vi "与工控机交互(子VI).vi"   [LabVIEW 2016, in "数据传输系统.lvlib"]
uses:
  <vilib>/ptbypt/NI_PtbyPt.lvlib
types:
  T1 = cluster{"setini":string, "sysini":string, "hechaini":string, "actualwrite":string, "actualread":string, "datasent":string, "反控命令信息队列":string, "反控与仪器交互":string}
  T2 = cluster{"仪器状态":u16[], "试剂余量":u16[], "各参数测量间隔":u16[], "关键参数":u16[], "校准点信息":u16[], "告警信息":u16[], "系统信息":u16[]}
  T3 = cluster{"[0]":bool, "[1]":bool, "[2]":bool, "[3]":bool, "[4]":bool}
  T4 = cluster{"[0]":bool, "[1]":bool, "[2]":bool, "[3]":bool, "[4]":bool, "[5]":bool}
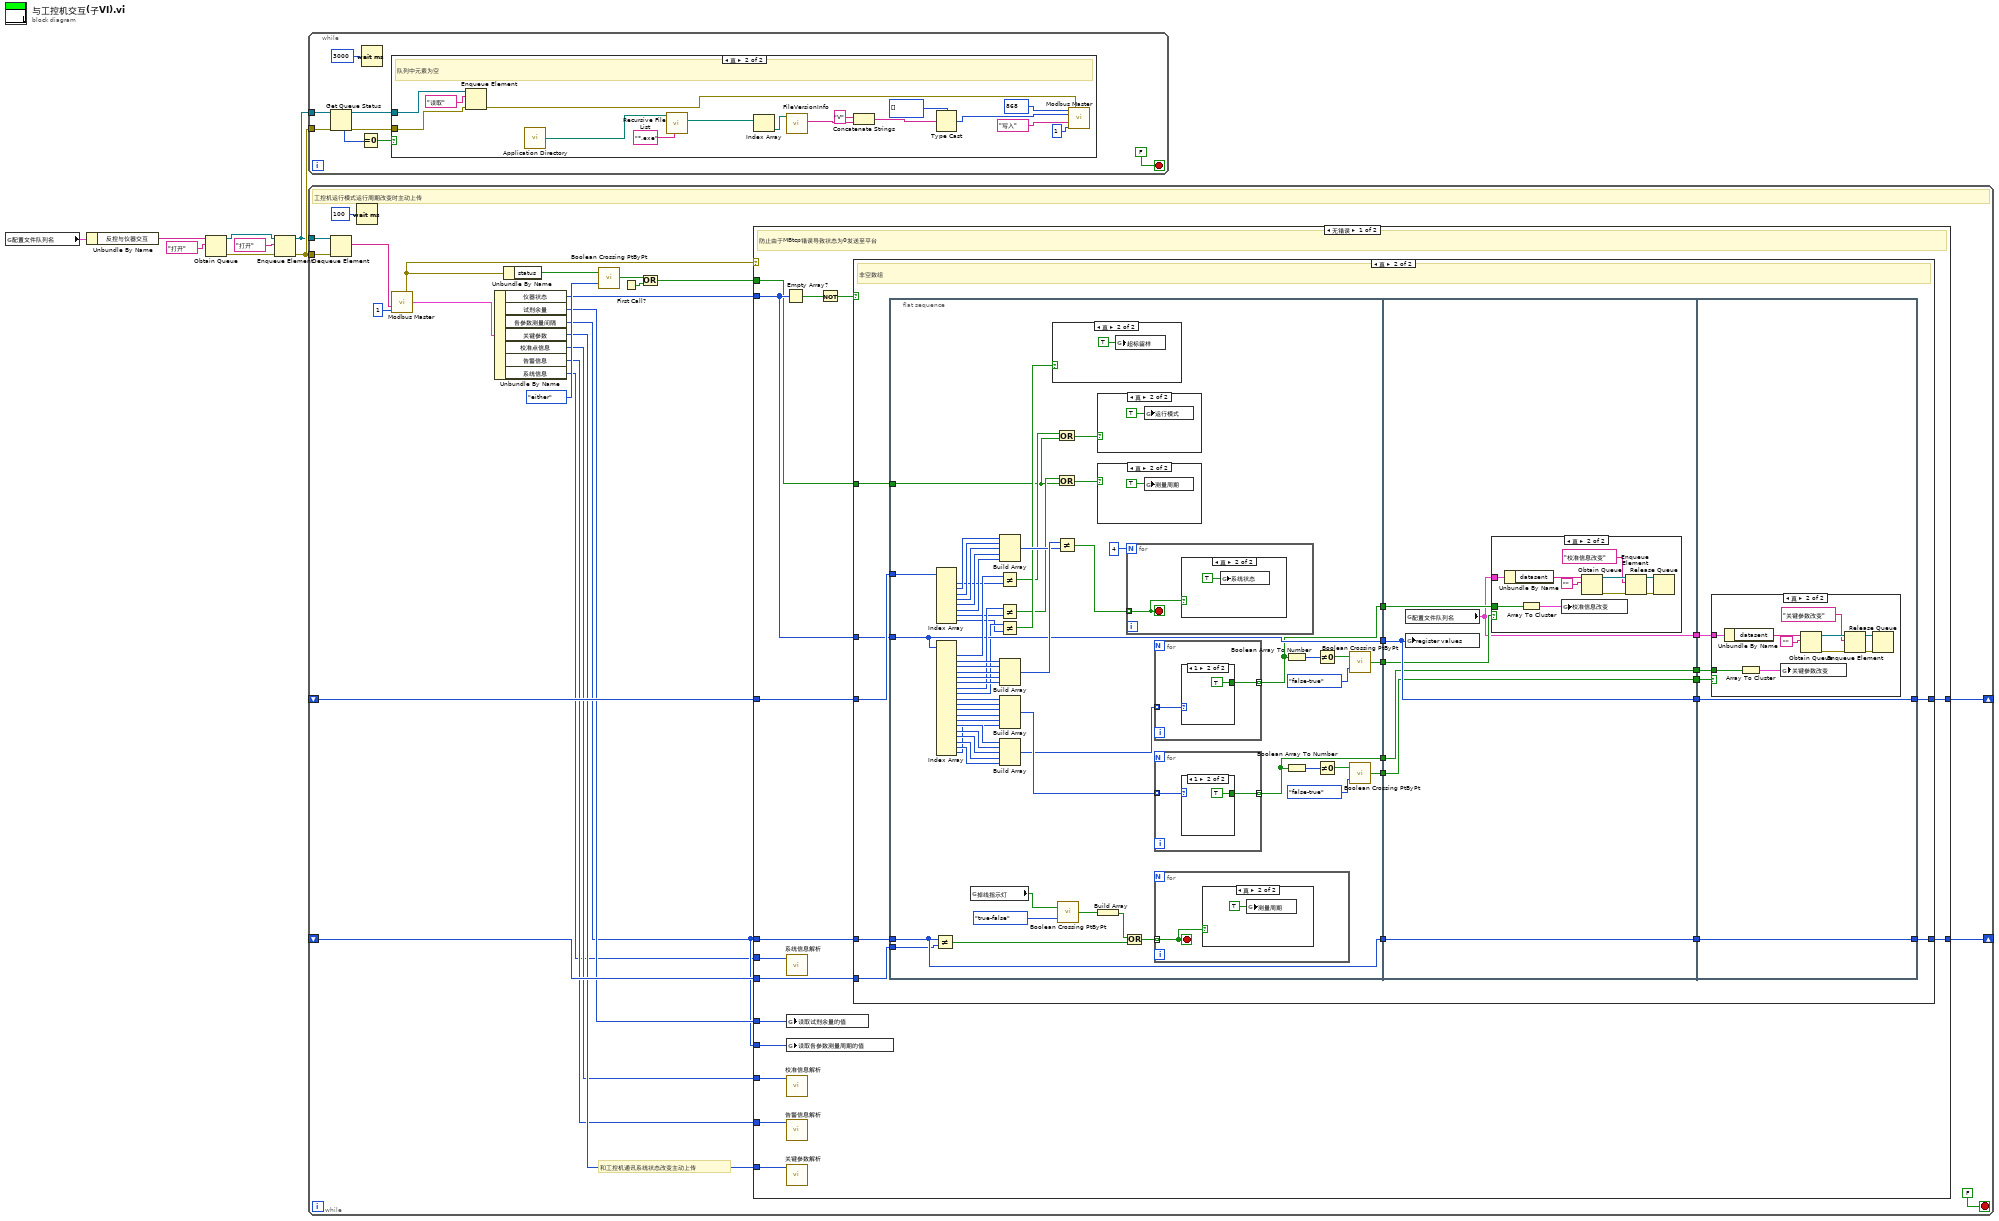
[diagram p0: block diagram]
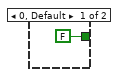
[diagram p4: hidden frame]
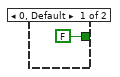
[diagram p5: hidden frame]
diagram:
  n1 = global read "全局1.vi" "配置文件队列名"() -> (w1:T1)
  n2 = Unbundle By Name(w1) -> ("反控与仪器交互"=w2:string)
  n3 = Obtain Queue(name (unnamed)=w2, element data type="打开" ("读取写入选择")) -> (queue out=w4:refnum<queue>, error out=w5:errorcluster)  [unwired: 3 in, 1 out]
  n4 = Enqueue Element(queue=w4, element="打开" ("读取写入选择"), error in (no error)=w5) -> (queue out=w6:refnum<queue>, error out=w7:errorcluster)  [unwired: 1 in, 1 out]
  n5 = while {
    tunnel: w6 -> [w13]
    tunnel: w7 -> [w12]
    stop <- FALSE stop-if-true
    n6 = Get Queue Status(queue=w13, error in (no error)=w12) -> (queue out=w10:refnum<queue>, error out=w9:errorcluster, # elements in queue=w14:i32)  [unwired: 1 in, 5 out]
    n7 = Equal To 0?(x=w14) -> (x = 0?=w11:bool)
    n8 = Wait (ms)(milliseconds to wait=u32 3000 ("等待时间（毫秒）")) -> ()  [unwired: 1 out]
    n9 = case shown="真" w11 {
      tunnel: w10 -> [_ w31]
      tunnel: w9 -> [_ w30]
      frame False {
      }
      frame True {
        # "队列中元素为空"
        n10 = Enqueue Element(queue=w31, element="读取" ("读取写入选择"), error in (no error)=w30) -> (error out=w26:errorcluster)  [unwired: 1 in, 2 out]
        n11 = call <vilib>:"Application Directory.vi"() -> ("Application Directory"=w24:path)
        n12 = call <vilib>:"Recursive File List.vi"("pattern"="*.exe", "Folder Path"=w24) -> ("All Files in Dir"=w22:path[])  [unwired: 5 in, 4 out]
        n13 = Index Array(array=w22) -> (element=w23:path)  [unwired: 1 in]
        n14 = call <vilib>:"FileVersionInfo.vi"("Application Path in"=w23) -> ("File Version Info"=w20:string)  [unwired: 7 in, 3 out]
        n15 = Concatenate Strings("V" ("字符串"), w20) -> (w18:string)
        n16 = Type Cast(type=u16[] [], x=w18) -> (*(type *) &x=w19:u16[])
        n17 = call "Modbus Master.vi"("starting address"=u16 868, "error in"=w26, "holding register values"=w19, "读取写入选择"="写入", "Unit ID"=u8 1) -> ()  [unwired: 4 in, 7 out]
      }
    }
  }
  n18 = while {
    tunnel: w6 -> [w53]
    tunnel: w7 -> [w52]
    shift-right: [w49] -> _
    shift-left: _ -> [w50]
    shift-right: [w42] -> _
    shift-left: _ -> [w41]
    stop <- FALSE stop-if-true
    # "和工控机通讯系统状态改变主动上传"
    # "工控机运行模式运行周期改变时主动上传"
    n19 = Dequeue Element(queue=w53, error in (no error)=w52) -> (element=w51:string)  [unwired: 1 in, 3 out]
    n20 = Wait (ms)(milliseconds to wait=u32 100 ("等待时间（毫秒）")) -> ()  [unwired: 1 out]
    n21 = call "Modbus Master.vi"("读取写入选择"=w51, "Unit ID"=u8 1) -> ("error out"=w48:errorcluster, "输出"=w40:T2)  [unwired: 7 in, 5 out]
    n22 = Unbundle By Name(w40) -> ("仪器状态"=w39:u16[], "试剂余量"=w38:u16[], "各参数测量间隔"=w37:u16[], "关键参数"=w36:u16[], "校准点信息"=w35:u16[], "告警信息"=w34:u16[], "系统信息"=w33:u16[])
    n23 = Unbundle By Name(w48) -> ("status"=w47:bool)
    n24 = call <vilib>:"Boolean Crossing PtByPt.vi"("direction"=enum16{"either", "false-true", "true-false"}."either", "input"=w47) -> ("crossing"=w45:bool)  [unwired: 1 in]
    n25 = First Call?() -> (First Call?: T/F=w44:bool)
    n26 = Or(x=w45, y=w44) -> (x .or. y?=w43:bool)
    n27 = case shown="无错误" w48 {
      tunnel: w39 -> [w69 _]
      tunnel: w50 -> [w71 w199]
      tunnel: [w70 w199] -> w49
      tunnel: w43 -> [w66 _]
      tunnel: w38 -> [w65 _]
      tunnel: w37 -> [w64 _]
      tunnel: w37 -> [w63 w198]
      tunnel: [w62 w198] -> w42
      tunnel: w41 -> [w61 _]
      tunnel: w36 -> [w60 _]
      tunnel: w35 -> [w59 _]
      tunnel: w34 -> [w58 _]
      tunnel: w33 -> [w57 _]
      frame No Error {
        # "防止由于MBtcp错误导致状态为0发送至平台"
        n28 = Empty Array?(array=w69) -> (empty?=w68:bool)
        n29 = call "系统信息解析.vi"("系统信息"=w57) -> ()  [unwired: 11 in]
        n30 = global write "全局1.vi" "读取试剂余量的值"(w65) -> ()
        n31 = global write "全局1.vi" "读取各参数测量周期的值"(w64) -> ()
        n32 = call "校准信息解析.vi"("校准信息"=w59) -> ()  [unwired: 11 in]
        n33 = call "告警信息解析.vi"("告警信息"=w58) -> ()  [unwired: 11 in]
        n34 = call "关键参数解析.vi"("关键参数"=w60) -> ()  [unwired: 11 in]
        n35 = Not(x=w68) -> (.not. x?=w67:bool)
        n36 = case shown="真" w67 {
          tunnel: w71 -> [w73 w90]
          tunnel: [w73 w89] -> w70
          tunnel: w69 -> [_ w88]
          tunnel: w66 -> [_ w87]
          tunnel: w63 -> [w72 w86]
          tunnel: [w72 w84] -> w62
          tunnel: w61 -> [_ w83]
          frame False {
          }
          frame True {
            # "非空数组"
            n37 = flat-sequence {
              tunnel: w88 -> [w134]
              tunnel: [w134] -> w91
              tunnel: w90 -> [w130]
              tunnel: w87 -> [w125]
              tunnel: w86 -> [w123]
              tunnel: [w123] -> w85
              tunnel: w83 -> [w122]
              tunnel: [w111] -> w82
              tunnel: [w100] -> w81
              tunnel: [w99] -> w80
              tunnel: [w98] -> w79
              tunnel: w91 -> [w172]
              tunnel: w85 -> [w171]
              tunnel: w82 -> [w167]
              tunnel: w81 -> [w170]
              tunnel: w80 -> [w169]
              tunnel: w79 -> [w168]
              tunnel: [w172] -> w78
              tunnel: [w171] -> w77
              tunnel: [w168] -> w76
              tunnel: [w167] -> w75
              tunnel: [w166] -> w74
              tunnel: [w186] -> w84
              tunnel: [w187] -> w89
              tunnel: w78 -> [w187]
              tunnel: w77 -> [w186]
              tunnel: w76 -> [w185]
              tunnel: w75 -> [w184]
              tunnel: w74 -> [w183]
              frame #0 {
                n38 = Not Equal?(x=w123, y=w122) -> (x != y?=w121:bool[])
                n39 = Index Array(array=w130) -> (element #1=w137:u16, element #2=w145:u16, element #3=w144:u16, element #4=w143:u16, element #5=w142:u16, element #6=w141:u16, element #7=w135:u16, element #8=w132:u16)  [unwired: 8 in]
                n40 = Index Array(array=w134) -> (element #1=w138:u16, element #2=w150:u16, element #3=w149:u16, element #4=w148:u16, element #5=w147:u16, element #6=w146:u16, element #7=w136:u16, element #8=w133:u16, element #9=w119:u16, element #10=w118:u16, element #11=w117:u16, element #12=w116:u16, element #13=w115:u16, element #14=w109:u16, element #15=w108:u16, element #16=w107:u16, element #17=w106:u16, element #18=w105:u16, element #19=w92:u16)  [unwired: 19 in]
                n41 = global read "全局 数据发送重叠.vi" "掉线指示灯"() -> (w96:bool)
                n42 = Not Equal?(x=w138, y=w137) -> (x != y?=w128:bool)
                n43 = Not Equal?(x=w136, y=w135) -> (x != y?=w126:bool)
                n44 = Not Equal?(x=w133, y=w132) -> (x != y?=w131:bool)
                n45 = Build Array(w145, w144, w143, w142, w141) -> (w139:u16[])
                n46 = Build Array(w150, w149, w148, w147, w146) -> (w140:u16[])
                n47 = Build Array(w119, w118, w117, w116, w115, w92) -> (w114:u16[])
                n48 = Build Array(w109, w108, w107, w106, w105) -> (w101:u16[])
                n49 = case shown="真" w131 {
                  frame False {
                  }
                  frame True {
                    n50 = global write "全局1.vi" "超标留样"(TRUE ("系统状态改变")) -> ()
                  }
                }
                n51 = Or(x=w128, y=w125) -> (x .or. y?=w127:bool)
                n52 = Or(x=w126, y=w125) -> (x .or. y?=w124:bool)
                n53 = Not Equal?(x=w140, y=w139) -> (x != y?=w129:bool[])
                n54 = call <vilib>:"Boolean Crossing PtByPt.vi"("direction"=enum16{"either", "false-true", "true-false"}."true-false", "input"=w96) -> ("crossing"=w94:bool)  [unwired: 1 in]
                n55 = case shown="真" w127 {
                  frame False {
                  }
                  frame True {
                    n56 = global write "全局1.vi" "运行模式"(TRUE) -> ()
                  }
                }
                n57 = case shown="真" w124 {
                  frame False {
                  }
                  frame True {
                    n58 = global write "全局1.vi" "测量周期"(TRUE ("系统状态改变")) -> ()
                  }
                }
                n59 = Build Array(w94) -> (w93:bool[])
                n60 = Or(x=w93, y=w121) -> (x .or. y?=w97:bool[])
                n61 = for {
                  N: 4 -> [_]
                  tunnel: w129 -> [w161] mode=indexing
                  stop <- w161 stop-if-true
                  n62 = case shown="真" w161 {
                    frame False {
                    }
                    frame True {
                      n63 = global write "全局1.vi" "系统状态"(TRUE ("系统状态改变")) -> ()
                    }
                  }
                }
                n64 = for {
                  tunnel: w101 -> [w152] mode=indexing
                  tunnel: [w151] -> w99 mode=indexing
                  n65 = case shown="1" w152 {
                    tunnel: [FALSE TRUE] -> w151
                    frame 0, Default {
                    }
                    frame 1 {
                    }
                  }
                }
                n66 = for {
                  tunnel: w114 -> [w156] mode=indexing
                  tunnel: [w155] -> w98 mode=indexing
                  n67 = case shown="1" w156 {
                    tunnel: [FALSE TRUE] -> w155
                    frame 0, Default {
                    }
                    frame 1 {
                    }
                  }
                }
                n68 = for {
                  tunnel: w97 -> [w159] mode=indexing
                  stop <- w159 stop-if-true
                  n69 = case shown="真" w159 {
                    frame False {
                    }
                    frame True {
                      n70 = global write "全局1.vi" "测量周期"(TRUE ("系统状态改变")) -> ()
                    }
                  }
                }
                n71 = Boolean Array To Number(Boolean array=w99) -> (number=w102:u32)
                n72 = Boolean Array To Number(Boolean array=w98) -> (number=w113:u32)
                n73 = Not Equal To 0?(x=w102) -> (x != 0?=w103:bool)
                n74 = Not Equal To 0?(x=w113) -> (x != 0?=w112:bool)
                n75 = call <vilib>:"Boolean Crossing PtByPt.vi"("direction"=enum16{"either", "false-true", "true-false"}."false-true", "input"=w103) -> ("crossing"=w100:bool)  [unwired: 1 in]
                n76 = call <vilib>:"Boolean Crossing PtByPt.vi"("direction"=enum16{"either", "false-true", "true-false"}."false-true", "input"=w112) -> ("crossing"=w111:bool)  [unwired: 1 in]
              }
              frame #1 {
                n77 = global read "全局1.vi" "配置文件队列名"() -> (w166:T1)
                n78 = global write "全局1.vi" "register values"(w172) -> ()
                n79 = case shown="真" w170 {
                  tunnel: w169 -> [_ w174]
                  tunnel: w166 -> [_ w173]
                  frame False {
                  }
                  frame True {
                    n80 = Unbundle By Name(w173) -> ("datasent"=w182:string)
                    n81 = Array To Cluster(array=w174) -> (cluster=w175:T3)
                    n82 = global write "全局1.vi" "校准信息改变"(w175) -> ()
                    n83 = Obtain Queue(name (unnamed)=w182, element data type="") -> (queue out=w180:refnum<queue>, error out=w178:errorcluster)  [unwired: 3 in, 1 out]
                    n84 = Enqueue Element(queue=w180, element="校准信息改变" ("元素"), error in (no error)=w178) -> (queue out=w177:refnum<queue>, error out=w176:errorcluster)  [unwired: 1 in, 1 out]
                    n85 = Release Queue(queue=w177, error in (no error)=w176) -> ()  [unwired: 1 in, 3 out]
                  }
                }
              }
              frame #2 {
                n86 = case shown="真" w184 {
                  tunnel: w185 -> [_ w189]
                  tunnel: w183 -> [_ w188]
                  frame False {
                  }
                  frame True {
                    n87 = Unbundle By Name(w188) -> ("datasent"=w197:string)
                    n88 = Array To Cluster(array=w189) -> (cluster=w190:T4)
                    n89 = global write "全局1.vi" "关键参数改变"(w190) -> ()
                    n90 = Obtain Queue(name (unnamed)=w197, element data type="") -> (queue out=w195:refnum<queue>, error out=w193:errorcluster)  [unwired: 3 in, 1 out]
                    n91 = Enqueue Element(queue=w195, element="关键参数改变" ("元素"), error in (no error)=w193) -> (queue out=w192:refnum<queue>, error out=w191:errorcluster)  [unwired: 1 in, 1 out]
                    n92 = Release Queue(queue=w192, error in (no error)=w191) -> ()  [unwired: 1 in, 3 out]
                  }
                }
              }
            }
          }
        }
      }
      frame Error {
      }
    }
  }
